vi "set scan from tracking.vi"(5 "init tracker":bool, 7 "tracking?":bool, 8 "counts per cycle":u16, 9 "tracking settings":T1, 10 "tracking state in":T3, 11 "scan specification":T2) -> (2 "tracking state out":T3, 3 "scan specification out":T2)   [LabVIEW 2010]
uses:
  kalman 3-axis state.ctl
  integrating single axis kalman state.ctl
  scan_specification_tagResonant.ctl
  polar tracking settings.ctl
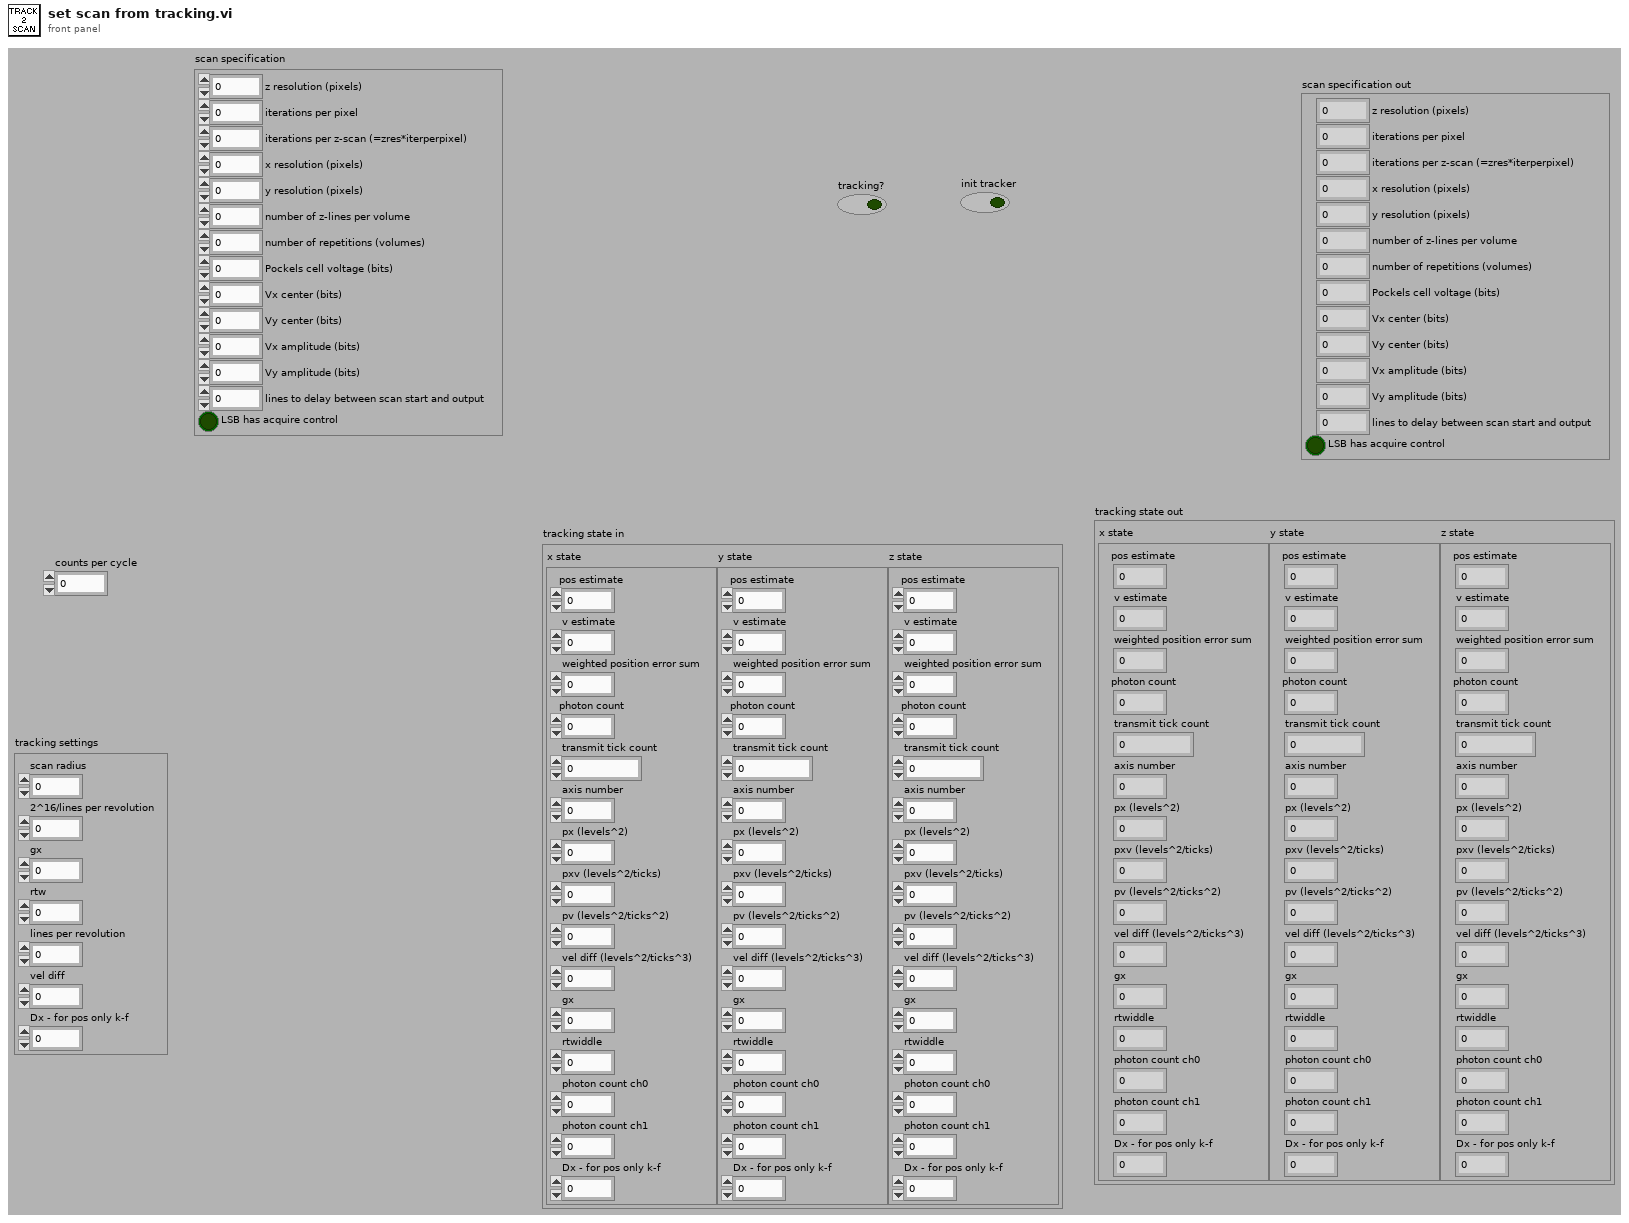
[diagram p1: front panel]
types:
  T1 = typedef "polar tracking settings.ctl" = cluster{"scan radius":u16, "2^16/lines per revolution":u16, "gx":fxp<+,16,8>, "rtw":fxp<+,16,26>, "lines per revolution":u8, "vel diff":fxp<+,24,-22>, "Dx - for pos only k-f":fxp<+,32,19>}
  T2 = typedef "scan_specification_tagResonant.ctl" = cluster{"z resolution (pixels)":u16, "iterations per pixel":u16, "iterations per z-scan (=zres*iterperpixel)":u16, "x resolution (pixels)":u16, "y resolution (pixels)":u16, "number of z-lines per volume":u16, "number of repetitions (volumes)":i32, "Pockels cell voltage (bits)":i16, "Vx center (bits)":i16, "Vy center (bits)":i16, "Vx amplitude (bits)":i16, "Vy amplitude (bits)":i16, "lines to delay between scan start and output":u16, "LSB has acquire control":bool}
  T3 = typedef "kalman 3-axis state.ctl" = cluster{"x state":T4, "y state":T4, "z state":T4}
  T4 = typedef "integrating single axis kalman state.ctl" = cluster{"pos estimate":fxp<+/-,32,16>, "v estimate":fxp<+/-,16,0>, "weighted position error sum":fxp<+/-,32,32>, "photon count":u32, "transmit tick count":u32, "axis number":u8, "px (levels^2)":fxp<+,32,19>, "pxv (levels^2/ticks)":fxp<+,32,2>, "pv (levels^2/ticks^2)":fxp<+,32,-14>, "vel diff (levels^2/ticks^3)":fxp<+,24,-22>, "gx":fxp<+,16,8>, "rtwiddle":fxp<+,16,26>, "photon count ch0":u32, "photon count ch1":u32, "Dx - for pos only k-f":fxp<+,32,19>}
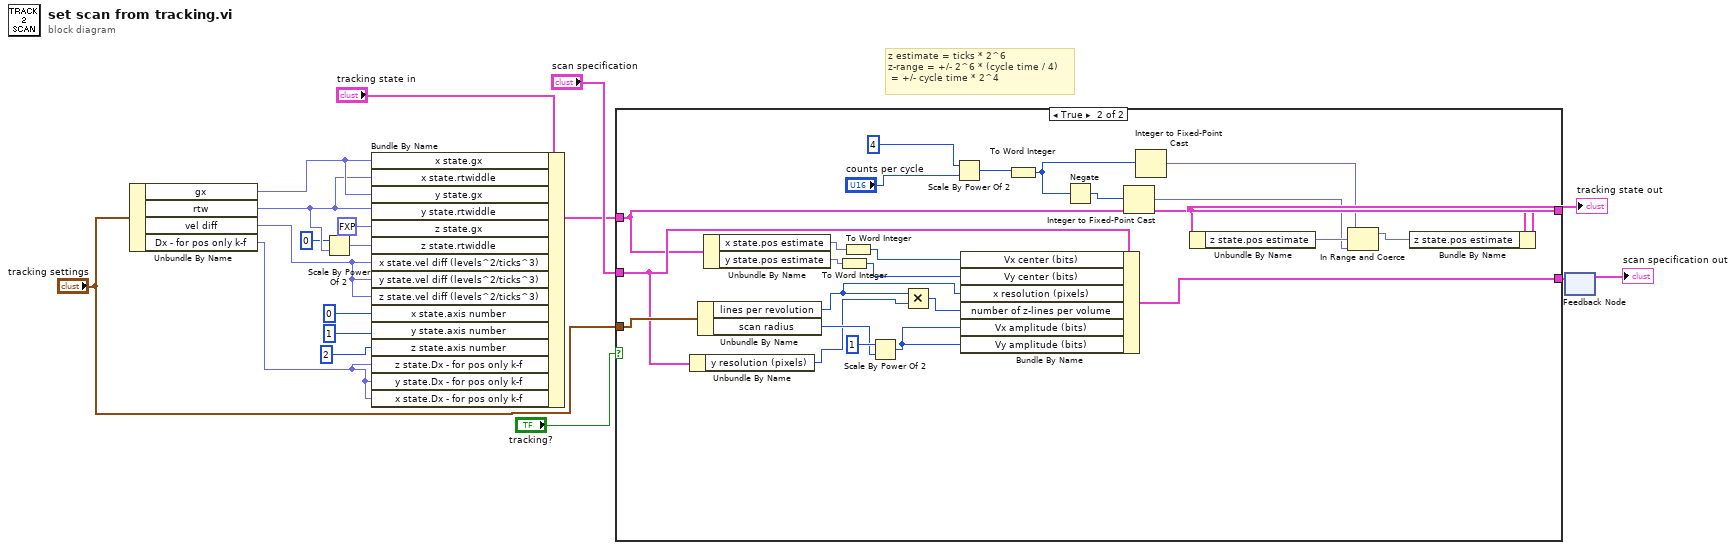
[diagram p0: block diagram]
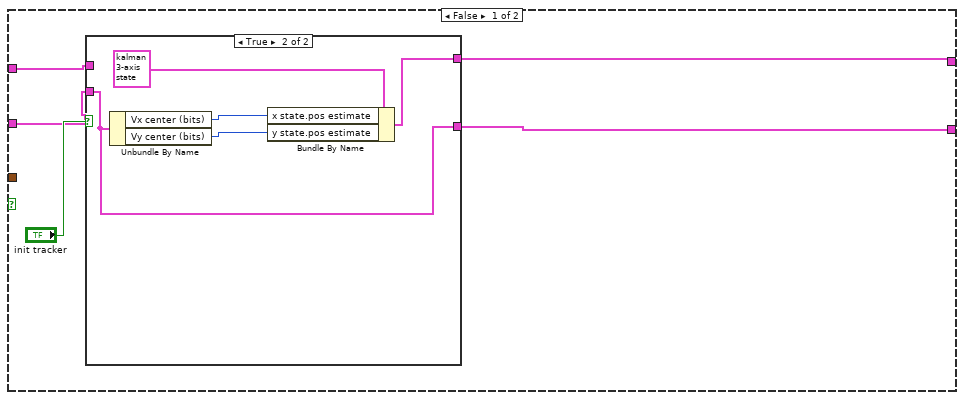
[diagram p2: hidden frame]
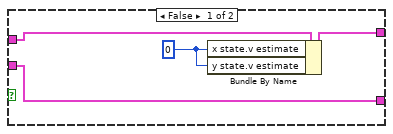
[diagram p3: hidden frame]
diagram:
  # "z estimate = ticks * 2^6\nz-range = +/- 2^6 * (cycle time / 4)\n = +/- cycle time * 2^4"
  n1 = Unbundle By Name("tracking settings") -> ("gx"=w10:fxp<+,16,8>, "rtw"=w8:fxp<+,16,26>, "vel diff"=w5:fxp<+,24,-22>, "Dx - for pos only k-f"=w1:fxp<+,32,19>)
  n2 = Scale By Power Of 2(n=0, x=w8) -> (x*2^n=w6:fxp<+,16,26>)
  n3 = Bundle By Name(cluster="tracking state in", "x state.gx"=w10, "x state.rtwiddle"=w8, "y state.gx"=w10, "y state.rtwiddle"=w8, "z state.gx"=fxp<+,16,8> 1.0, "z state.rtwiddle"=w6, "x state.vel diff (levels^2/ticks^3)"=w5, "y state.vel diff (levels^2/ticks^3)"=w5, "z state.vel diff (levels^2/ticks^3)"=w5, "x state.axis number"=u8 0 ("x state.axes number"), "y state.axis number"=u8 1 ("y state.axes number"), "z state.axis number"=u8 2 ("z state.axes number"), "z state.Dx - for pos only k-f"=w1, "y state.Dx - for pos only k-f"=w1, "x state.Dx - for pos only k-f"=w1) -> (w12:T3)
  n4 = case shown="True" "tracking?" {
    tunnel: w12 -> [w22 w43]
    tunnel: "scan specification" -> [w21 w47]
    tunnel: [w19 w34] -> w16
    tunnel: [w20 w54] -> w15
    tunnel: "tracking settings" -> [_ w49]
    frame False {
      n5 = case shown="True" "init tracker" {
        tunnel: w22 -> [w26 _]
        tunnel: w21 -> [w27 w32]
        tunnel: [w25 w28] -> w19
        tunnel: [w27 w32] -> w20
        frame False {
          w24 = i16 0
          n6 = Bundle By Name(cluster=w26, "x state.v estimate"=w24, "y state.v estimate"=w24) -> (w25:T3)
        }
        frame True {
          n7 = Unbundle By Name(w32) -> ("Vx center (bits)"=w30:i16, "Vy center (bits)"=w29:i16)
          n8 = Bundle By Name(cluster=T3 {"x state"={"pos estimate"=0.0, "v estimate"=0.0, "weighted position error sum"=0.0, "photon count"=0, "transmit tick count"=0, "axis number"=0, "px (levels^2)"=0.0, "pxv (levels^2/ticks)"=0.0, "pv (levels^2/ticks^2)"=0.0, "vel diff (levels^2/ticks^3)"=0.0, "gx"=0.0, "rtwiddle"=0.0, "photon count ch0"=0, "photon count ch1"=0, "Dx - for pos only k-f"=0.0}, "y state"={"pos estimate"=0.0, "v estimate"=0.0, "weighted position error sum"=0.0, "photon count"=0, "transmit tick count"=0, "axis number"=1, "px (levels^2)"=0.0, "pxv (levels^2/ticks)"=0.0, "pv (levels^2/ticks^2)"=0.0, "vel diff (levels^2/ticks^3)"=0.0, "gx"=0.0, "rtwiddle"=0.0, "photon count ch0"=0, "photon count ch1"=0, "Dx - for pos only k-f"=0.0}, "z state"={"pos estimate"=0.0, "v estimate"=0.0, "weighted position error sum"=0.0, "photon count"=0, "transmit tick count"=0, "axis number"=2, "px (levels^2)"=0.0, "pxv (levels^2/ticks)"=0.0, "pv (levels^2/ticks^2)"=0.0, "vel diff (levels^2/ticks^3)"=0.0, "gx"=0.0, "rtwiddle"=0.0, "photon count ch0"=0, "photon count ch1"=0, "Dx - for pos only k-f"=0.0}} ("tracking state in"), "x state.pos estimate"=w30, "y state.pos estimate"=w29) -> (w28:T3)
        }
      }
    }
    frame True {
      n9 = Unbundle By Name(w47) -> ("y resolution (pixels)"=w46:u16)
      n10 = Unbundle By Name(w49) -> ("lines per revolution"=w44:u8, "scan radius"=w48:u16)
      n11 = Unbundle By Name(w43) -> ("x state.pos estimate"=w53:fxp<+/-,32,16>, "y state.pos estimate"=w51:fxp<+/-,32,16>)
      n12 = To Word Integer(number=w51) -> (16bit integer=w50:i16)
      n13 = To Word Integer(number=w53) -> (16bit integer=w52:i16)
      n14 = Scale By Power Of 2(n=1, x=w48) -> (x*2^n=w55:u16)
      n15 = Multiply(x=w44, y=w46) -> (x*y=w45:u16)
      n16 = Scale By Power Of 2(n=u8 4 ("x"), x="counts per cycle") -> (x*2^n=w41:u16)
      n17 = Bundle By Name(cluster=w47, "Vx center (bits)"=w52, "Vy center (bits)"=w50, "x resolution (pixels)"=w44, "number of z-lines per volume"=w45, "Vx amplitude (bits)"=w55, "Vy amplitude (bits)"=w55) -> (w54:T2)
      n18 = To Word Integer(number=w41) -> (16bit integer=w38:i16)
      n19 = Negate(x=w38) -> (-x=w37:i16)
      n20 = Integer to Fixed-Point Cast(integer=w37) -> (fixed-point=w36:fxp<+/-,16,16>)  [unwired: 1 in]
      n21 = Integer to Fixed-Point Cast(integer=w38) -> (fixed-point=w35:fxp<+/-,16,16>)  [unwired: 1 in]
      n22 = Unbundle By Name(w43) -> ("z state.pos estimate"=w42:fxp<+/-,32,16>)
      n23 = In Range and Coerce(upper limit=w35, x=w42, lower limit=w36) -> (coerced(x)=w33:fxp<+/-,32,16>)  [unwired: 1 out]
      n24 = Bundle By Name(cluster=w43, "z state.pos estimate"=w33) -> (w34:T3)
    }
  }
  "tracking state out" <- w16
  n25 = feedback-in #1(w15) -> ()
  n26 = feedback #1() -> (→"scan specification out":T2)  [unwired: 1 in]
